vi "WildDrive_v2.vi"(9 "Super Turn":bool, 10 "Turn":dbl, 11 "Speed":dbl) -> (2 "Right Side Power":dbl, 3 "Left Side Power":dbl)   [LabVIEW 2018]
panel:
  in  "Manual Feed Forward (speed)":dbl=0.2
  in  "Manual Feed Forward (turn)":dbl=0.1
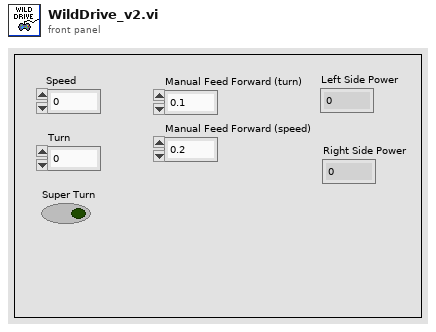
[diagram p1: front panel]
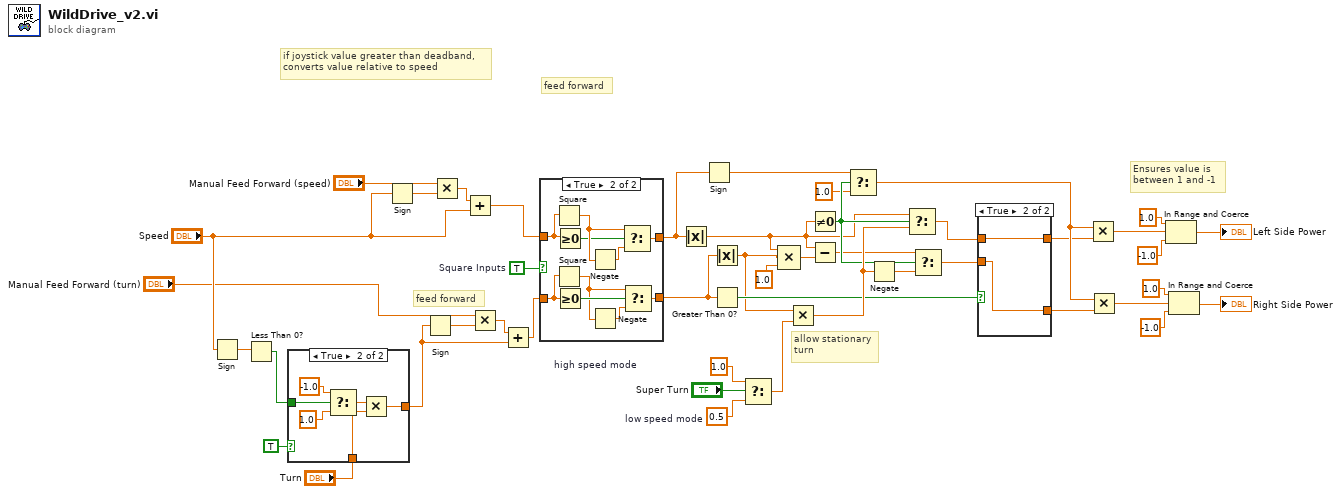
[diagram p0: block diagram]
diagram:
  w44 = 0.5  # low speed mode
  w43 = 1.0  # high speed mode
  w21 = TRUE  # Square Inputs
  # "feed forward"
  # "feed forward"
  # "Ensures value is \nbetween 1 and -1"
  # "if joystick value greater than deadband,\nconverts value relative to speed"
  # "allow stationary\nturn"
  n1 = Sign(1:"Speed") -> (0:w12:dbl)
  n2 = Less Than 0?(x=w12) -> (x < 0?=w14:bool)
  n3 = case shown="True" TRUE {
    tunnel: w14 -> [_ w51]
    tunnel: [w46 w48] -> w13
    tunnel: "Turn" -> [w46 w47]
    frame False {
    }
    frame True {
      n4 = Select(t=-1.0, s=w51, f=1.0) -> (s? t:f=w52:dbl)
      n5 = Multiply(x=w52, y=w47) -> (x*y=w48:dbl)
    }
  }
  n6 = Sign(1:"Speed") -> (0:w7:dbl)
  n7 = Sign(1:w13) -> (0:w15:dbl)
  n8 = Multiply(x="Manual Feed Forward (speed)", y=w7) -> (x*y=w8:dbl)
  n9 = Add(x=w8, y="Speed") -> (x+y=w6:dbl)
  n10 = Multiply(x="Manual Feed Forward (turn)", y=w15) -> (x*y=w16:dbl)
  n11 = Add(x=w16, y=w13) -> (x+y=w17:dbl)
  n12 = case shown="True" w21 {
    tunnel: [w53 w64] -> w19
    tunnel: [w54 w63] -> w18
    tunnel: w17 -> [w53 w62]
    tunnel: w6 -> [w54 w61]
    frame False {
    }
    frame True {
      n13 = Square(x=w61) -> (x^2=w56:dbl)
      n14 = Square(x=w62) -> (x^2=w59:dbl)
      n15 = Greater Or Equal To 0?(x=w61) -> (x >= 0?=w55:bool)
      n16 = Greater Or Equal To 0?(x=w62) -> (x >= 0?=w60:bool)
      n17 = Negate(x=w56) -> (-x=w57:dbl)
      n18 = Negate(x=w59) -> (-x=w58:dbl)
      n19 = Select(t=w56, s=w55, f=w57) -> (s? t:f=w63:dbl)
      n20 = Select(t=w59, s=w60, f=w58) -> (s? t:f=w64:dbl)
    }
  }
  n21 = Absolute Value(x=w18) -> (abs(x)=w1:dbl)
  n22 = Sign(1:w18) -> (0:w22:dbl)
  n23 = Absolute Value(x=w19) -> (abs(x)=w3:dbl)
  n24 = Greater Than 0?(x=w19) -> (x > 0?=w20:bool)
  n25 = Select(t=w43, s="Super Turn", f=w44) -> (s? t:f=w45:dbl)
  n26 = Compound Arithmetic op=MULTIPLY(w1, w3, 1.0 ("y")) -> (w24:dbl)
  n27 = Multiply(x=w3, y=w45) -> (x*y=w29:dbl)
  n28 = Not Equal To 0?(x=w1) -> (x != 0?=w28:bool)
  n29 = Subtract(x=w1, y=w24) -> (x-y=w26:dbl)
  n30 = Select(t=w22, s=w28, f=1.0) -> (s? t:f=w38:dbl)
  n31 = Negate(x=w29) -> (-x=w30:dbl)
  n32 = Select(t=w1, s=w28, f=w29) -> (s? t:f=w27:dbl)
  n33 = Select(t=w26, s=w28, f=w30) -> (s? t:f=w25:dbl)
  n34 = case shown="True" w20 {
    tunnel: w25 -> [w65 w68]
    tunnel: [w65 w67] -> w37
    tunnel: w27 -> [w66 w67]
    tunnel: [w66 w68] -> w39
    frame False {
    }
    frame True {
    }
  }
  n35 = Multiply(x=w38, y=w37) -> (x*y=w31:dbl)
  n36 = Multiply(x=w38, y=w39) -> (x*y=w36:dbl)
  n37 = In Range and Coerce(upper limit=1.0, x=w31, lower limit=-1.0) -> (coerced(x)=→"Left Side Power":dbl)  [unwired: 1 out]
  n38 = In Range and Coerce(upper limit=1.0, x=w36, lower limit=-1.0) -> (coerced(x)=→"Right Side Power":dbl)  [unwired: 1 out]
